vi "Triangular Moments.vi"(8 "xmax":dbl=1.0, 9 "xmode":dbl=nan, 10 "xmin":dbl) -> (0 "error":i32, 2 "variance":dbl=1.0, 3 "mean":dbl)   [LabVIEW 2024, in "NI_Gmath.lvlib"]
doc: "<p>Returns the expected mean and variance of the random variate <em>X</em>, where <em>X</em> describes the selected distribution type. You must <a href=\"nihelplauncher://docs/csh?context=lvcore_lvhowto_selectingdefaultinstpolyvi\">manually select the polymorphic instance</a> to use.</p>"
uses:
  NI_Gmath.lvlib
  st_error_code.ctl
panel:
  # "Triangular Moments"
  # "NaN maps to \n(xmax-xmin)/2"
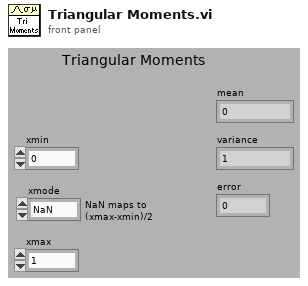
[diagram p1: front panel]
types:
  T1 = typedef "NI_Gmath.lvlib/st_error_code.ctl" = i32
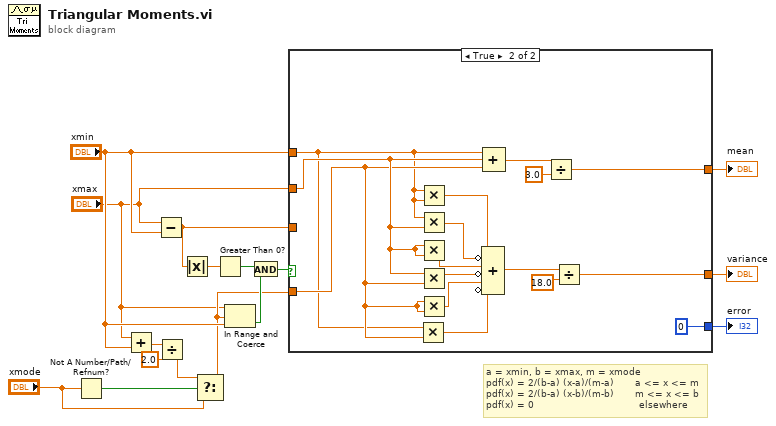
[diagram p0: block diagram]
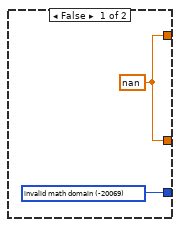
[diagram p2: hidden frame]
diagram:
  # "a = xmin, b = xmax, m = xmode\npdf(x) = 2/(b-a) (x-a)/(m-a)       a <= x <= m\npdf(x) = 2/(b-a) (x-b)/(m-b)       m <= x <= b\npdf(x) = 0                                   elsewhere"
  n1 = Not A Number/Path/Refnum?(number/path/refnum="xmode") -> (NaN/Path/Refnum?=w6:bool)
  n2 = Add(x="xmax", y="xmin") -> (x+y=w9:dbl)
  n3 = Subtract(x="xmax", y="xmin") -> (x-y=w11:dbl)
  n4 = Divide(x=w9, y=2.0) -> (x/y=w7:dbl)
  n5 = Absolute Value(x=w11) -> (abs(x)=w16:dbl)
  n6 = Select(t=w7, s=w6, f="xmode") -> (s? t:f=w3:dbl)
  n7 = Greater Than 0?(x=w16) -> (x > 0?=w13:bool)
  n8 = In Range and Coerce(upper limit="xmax", x=w3, lower limit="xmin") -> (In Range?=w4:bool)  [unwired: 1 out]
  n9 = And(x=w13, y=w4) -> (x .and. y?=w12:bool)
  n10 = case shown="True" w12 {
    tunnel: "xmin" -> [_ w28]
    tunnel: w11 -> [_ _]
    tunnel: [w18 w31] -> w15
    tunnel: [w17 0] -> w14
    tunnel: w3 -> [_ w29]
    tunnel: "xmax" -> [_ w30]
    tunnel: [w18 w20] -> w1
    frame False {
      w17 = T1 -20069 items=["invalid math domain"=-20069, "Fourier interpolation size m >= n"=-20070, "empty array"=-20003] ("stat interp error code")
      w18 = nan
    }
    frame True {
      n11 = Multiply(x=w28, y=w29) -> (x*y=w24:dbl)
      n12 = Multiply(x=w28, y=w28) -> (x*y=w27:dbl)
      n13 = Multiply(x=w28, y=w30) -> (x*y=w22:dbl)
      n14 = Multiply(x=w30, y=w30) -> (x*y=w26:dbl)
      n15 = Multiply(x=w30, y=w29) -> (x*y=w23:dbl)
      n16 = Multiply(x=w29, y=w29) -> (x*y=w25:dbl)
      n17 = Compound Arithmetic op=ADD(w27, invert w22, w26, invert w23, w25, invert w24) -> (w19:dbl)
      n18 = Compound Arithmetic op=ADD(w28, w30, w29) -> (w32:dbl)
      n19 = Divide(x=w32, y=3.0) -> (x/y=w31:dbl)
      n20 = Divide(x=w19, y=18.0) -> (x/y=w20:dbl)
    }
  }
  "mean" <- w15
  "error" <- w14
  "variance" <- w1
